vi "Eval Condition.vi"(7 "Variables":refnum<class "Variables.lvclass">, 8 "error in (no error)":errorcluster, 9 "Sequence Time":T1, 11 "HighLimit Condition in":refnum<class "HighLimit Condition.lvclass">) -> (0 "error out":errorcluster, 2 "Result":bool, 3 "HighLimit Condition out":refnum<class "HighLimit Condition.lvclass">)   [LabVIEW 2020, in "VolatusSeq.lvlib" / "HighLimit Condition.lvclass"]
uses:
  HighLimit Condition.lvclass
  Sequence Time.ctl
  Variables/Variables.lvclass
  HighLimit Condition.lvclass/HighLimit Condition.ctl
  lv-vecto/Vecto/Channel DBL/Channel DBL.lvclass/Channel DBL.ctl
  lv-vecto/Vecto/Group DBL/Value by Index.vi
  Condition Value/Condition Value.lvclass
  VolatusSeq.lvlib
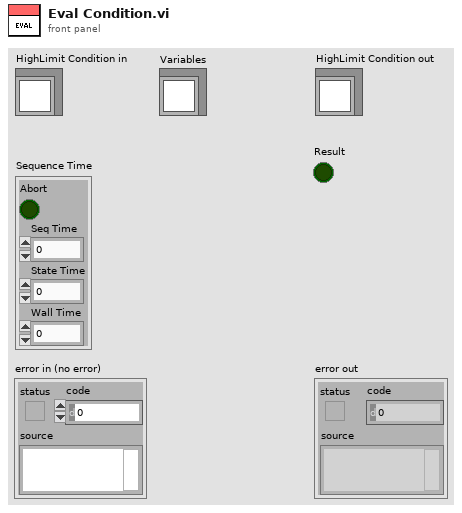
[diagram p1: front panel]
types:
  T1 = typedef "VolatusSeq.lvlib/Sequence Time.ctl" = cluster{"Abort":bool, "Seq Time":dbl, "State Time":dbl, "Wall Time":dbl}
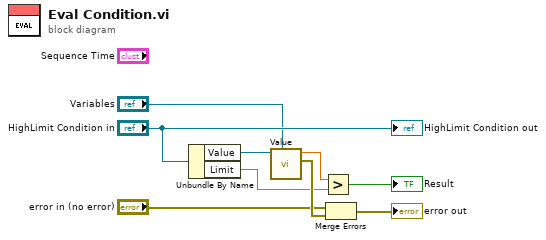
[diagram p0: block diagram]
diagram:
  n1 = Unbundle By Name("HighLimit Condition in") -> ("Value"=w6:refnum<class "Condition Value.lvclass">, "Limit"=w4:dbl)
  n2 = call "Value.vi"("Variables"="Variables", "Condition Value in"=w6) -> ("error out"=w9:errorcluster, "Value"=w5:dbl)  [unwired: 8 in]
  n3 = Greater?(x=w5, y=w4) -> (0:→"Result":bool)
  n4 = Merge Errors("error in (no error)", w9) -> (→"error out":errorcluster)
  "HighLimit Condition out" <- "HighLimit Condition in"
